vi "Get Inverse Kinematics Matrix.vi"(11 "Radii (ft)":T1 {"Right Back Position" format="%.2f"; "Right Front Position" format="%.2f"; "Left Back Position" format="%.2f"; "Left Front Position" format="%.2f"}) -> (3 "Real Matrix":T2)   [LabVIEW 2020]
uses:
  <vilib>/Analysis/Matrix/Datatypes/RealMatrix.ctl
  Type Definitions/Data/Pod Positions.ctl
  <vilib>/Analysis/Matrix/NI_Matrix.lvlib
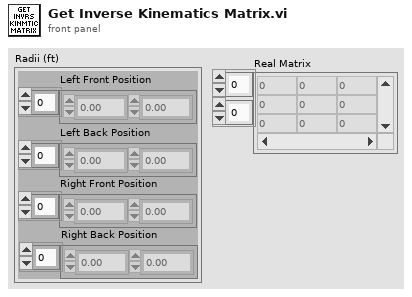
[diagram p1: front panel]
types:
  T1 = typedef "Pod Positions.ctl" = cluster{"Left Front Position":dbl[], "Left Back Position":dbl[], "Right Front Position":dbl[], "Right Back Position":dbl[]}
  T2 = typedef "NI_Matrix.lvlib/RealMatrix.ctl" = dbl[][]
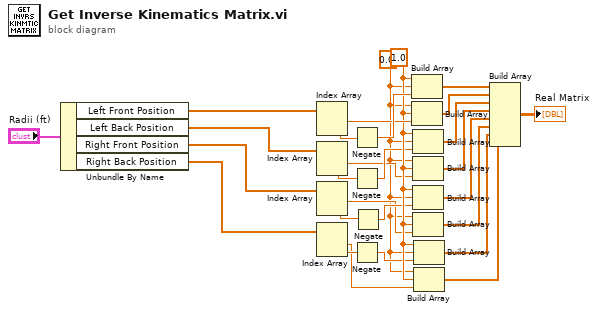
[diagram p0: block diagram]
diagram:
  w6 = 0.0 ("element")
  w20 = 1.0 ("element")
  n1 = Unbundle By Name("Radii (ft)") -> ("Left Front Position"=w4:dbl[], "Left Back Position"=w3:dbl[], "Right Front Position"=w2:dbl[], "Right Back Position"=w1:dbl[])
  n2 = Index Array(array=w4) -> (element #1=w22:dbl, element #2=w27:dbl)  [unwired: 2 in]
  n3 = Index Array(array=w3) -> (element #1=w18:dbl, element #2=w17:dbl)  [unwired: 2 in]
  n4 = Index Array(array=w2) -> (element #1=w15:dbl, element #2=w26:dbl)  [unwired: 2 in]
  n5 = Index Array(array=w1) -> (element #1=w13:dbl, element #2=w25:dbl)  [unwired: 2 in]
  n6 = Negate(x=w27) -> (-x=w24:dbl)
  n7 = Negate(x=w17) -> (-x=w19:dbl)
  n8 = Negate(x=w25) -> (-x=w14:dbl)
  n9 = Negate(x=w26) -> (-x=w16:dbl)
  n10 = Build Array(w20, w6, w24) -> (w23:dbl[])
  n11 = Build Array(w6, w20, w22) -> (w21:dbl[])
  n12 = Build Array(w20, w6, w19) -> (w12:dbl[])
  n13 = Build Array(w6, w20, w18) -> (w11:dbl[])
  n14 = Build Array(w20, w6, w16) -> (w10:dbl[])
  n15 = Build Array(w6, w20, w15) -> (w9:dbl[])
  n16 = Build Array(w20, w6, w14) -> (w8:dbl[])
  n17 = Build Array(w6, w20, w13) -> (w7:dbl[])
  n18 = Build Array(w23, w21, w12, w11, w10, w9, w8, w7) -> (→"Real Matrix":T2)
